vi "Get PS Status.vi"(8 "error in (no error)":errorcluster, 10 "Status":variant, 11 "PS Driver.lvlib:PS Driver.lvclass":refnum<class "PS Driver.lvclass">) -> (0 "error out":errorcluster, 2 "Status out":variant, 3 "PS Driver.lvlib:PS Driver.lvclass out":refnum<class "PS Driver.lvclass">)   [LabVIEW 2019, in "PS Driver.lvlib" / "PS Driver.lvclass"]
uses:
  PS Driver.lvclass
  PS Driver.lvclass/PS Driver.ctl
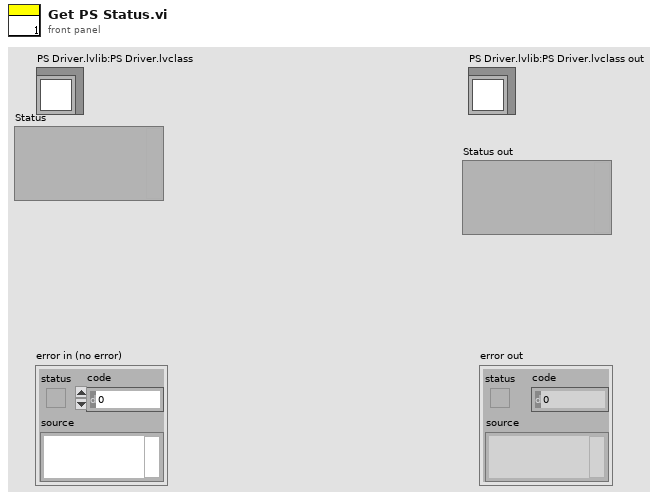
[diagram p1: front panel]
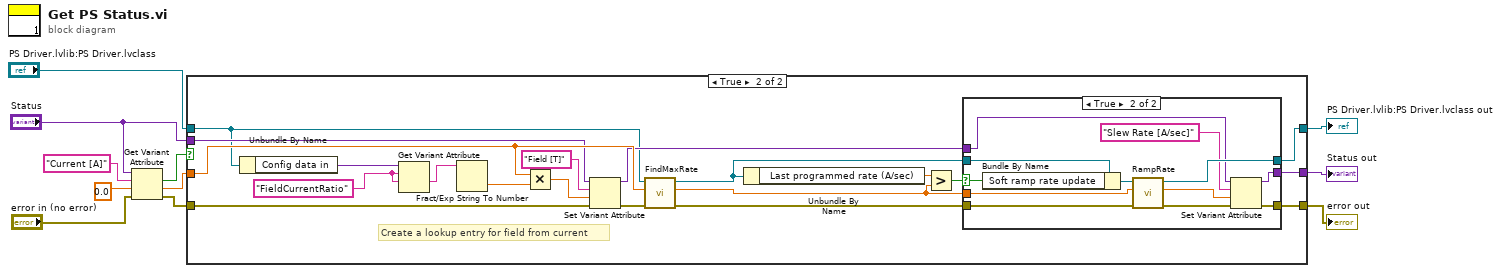
[diagram p0: block diagram]
diagram:
  n1 = Get Variant Attribute(Variant="Status", name="Current [A]", default value (empty Variant)=0.0, error in="error in (no error)") -> (found=w9:bool, value=w8:dbl, error out=w5:errorcluster)  [unwired: 1 out]
  n2 = case shown="True" w9 {
    tunnel: w8 -> [_ w26]
    tunnel: "PS Driver.lvlib:PS Driver.lvclass" -> [w14 w19]
    tunnel: [w13 w29] -> w6
    tunnel: w5 -> [w13 w20]
    tunnel: [w14 w28] -> w4
    tunnel: "Status" -> [w12 w24]
    tunnel: [w12 w27] -> w2
    frame False {
    }
    frame True {
      w16 = "FieldCurrentRatio" ("name")
      # "Create a lookup entry for field from current"
      n3 = Unbundle By Name(w19) -> ("Config data in"=w17:variant)
      n4 = Get Variant Attribute(Variant=w17, name=w16, default value (empty Variant)=w16) -> (value=w18:string)  [unwired: 1 in, 3 out]
      n5 = Fract/Exp String To Number(string=w18) -> (number=w15:dbl)  [unwired: 3 in, 1 out]
      n6 = Multiply(x=w26, y=w15) -> (x*y=w22:dbl)
      n7 = Set Variant Attribute(Variant=w24, name="Field [T]", value=w22, error in=w20) -> (Variant out=w25:variant, error out=w21:errorcluster)  [unwired: 1 out]
      n8 = call "FindMaxRate.vi"("error in (no error)"=w21, "Current (A)"=w26, "PS Driver in"=w19) -> ("error out"=w30:errorcluster, "Max rate (A/sec)"=w31:dbl, "PS Driver out"=w32:refnum<class "PS Driver.lvclass">)  [unwired: 6 in]
      n9 = Unbundle By Name(w32) -> ("Last programmed rate (A/sec)"=w34:dbl)
      n10 = Greater?(x=w34, y=w31) -> (0:w33:bool)
      n11 = case shown="True" w33 {
        selector: w33 -> [_ w48]
        tunnel: w32 -> [w37 w49]
        tunnel: w31 -> [_ w47]
        tunnel: w30 -> [w36 w46]
        tunnel: [w36 w40] -> w29
        tunnel: [w37 w44] -> w28
        tunnel: w25 -> [w35 w43]
        tunnel: [w35 w39] -> w27
        frame False {
        }
        frame True {
          n12 = Bundle By Name(cluster=w49, "Soft ramp rate update"=w48) -> (w45:refnum<class "PS Driver.lvclass">)
          n13 = call-dynamic "RampRate.vi"("error in (no error)"=w46, "Ramp rate (A/sec)"=w47, "PS Driver in"=w45) -> ("error out"=w41:errorcluster, "Ramp rate out (A/s)"=w38:dbl, "PS Driver out"=w44:refnum<class "PS Driver.lvclass">)  [unwired: 6 in]
          n14 = Set Variant Attribute(Variant=w43, name="Slew Rate [A/sec]", value=w38, error in=w41) -> (Variant out=w39:variant, error out=w40:errorcluster)  [unwired: 1 out]
        }
      }
    }
  }
  "error out" <- w6
  "PS Driver.lvlib:PS Driver.lvclass out" <- w4
  "Status out" <- w2
